vi "UserErrorHandle.vi"(8 "错误输入":errorcluster caption="错误输入（无错误）", 9 "错误解释":string="请检查串口连接和COM号是否正确", 10 "错误源":string="开关量模块", 11 "错误编号":i32=-8001) -> (0 "错误输出":errorcluster)   [LabVIEW 2018]
uses:
  <vilib>/Utility/error.llb/DialogType.ctl
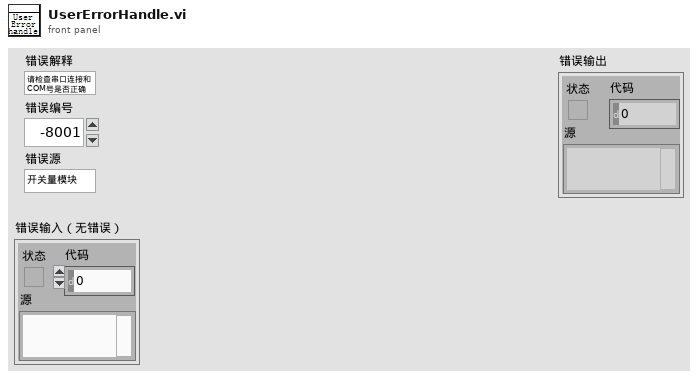
[diagram p1: front panel]
types:
  T1 = typedef "DialogType.ctl" = u16
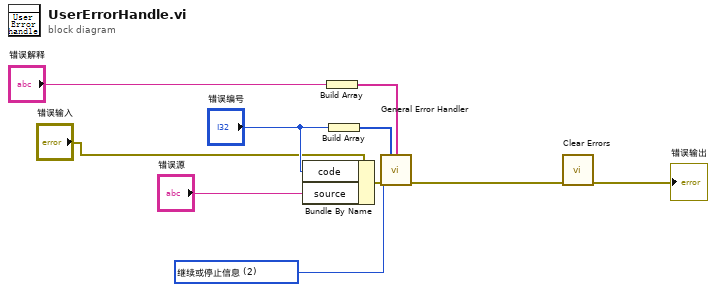
[diagram p0: block diagram]
diagram:
  w1 = T1 2 items=["无对话框", "确定信息", "继续或停止信息", "确定信息＋警告", "继续/停止+警告"] ("type of dialog (OK msg:1)")
  n1 = Bundle By Name(cluster="错误输入", "code"="错误编号", "source"="错误源") -> (w5:errorcluster)
  n2 = Build Array("错误解释") -> (w7:string[])
  n3 = Build Array("错误编号") -> (w8:i32[])
  n4 = call <vilib>:"General Error Handler.vi"("[user-defined codes]"=w8, "[user-defined descriptions]"=w7, "type of dialog (OK msg:1)"=w1, "error in (no error)"=w5) -> ("error out"=w6:errorcluster)  [unwired: 7 in, 4 out]
  n5 = call <vilib>:"Clear Errors.vi"("error in (no error)"=w6) -> ("error out"=→"错误输出":errorcluster)  [unwired: 5 in, 1 out]
